vi "Test Elapsed Time.vi"() -> ()   [LabVIEW 2021, in "Interval Timer.lvlib"]
uses:
  Interval Timer.lvlib
panel:
  out "elapsed time (s)":dbl
  out "start time":timestamp
  out "current time":timestamp
  in  "wait (ms)":dbl=1000.0
  in  "reset?":bool
  in  "stop":bool
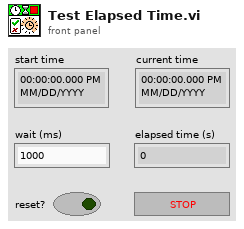
[diagram p1: front panel]
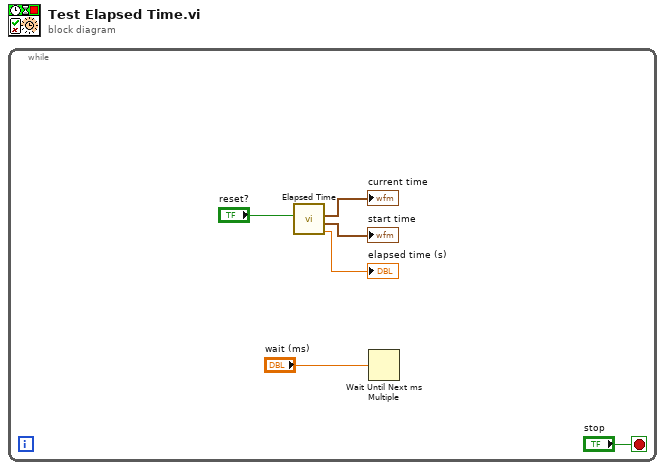
[diagram p0: block diagram]
diagram:
  n1 = while {
    stop <- "stop" stop-if-true
    n2 = call "Elapsed Time.vi"("reset timer"="reset?") -> ("elapsed time (s)"=→"elapsed time (s)":dbl, "start time"=→"start time":timestamp, "current time"=→"current time":timestamp)  [unwired: 8 in]
    n3 = Wait Until Next ms Multiple(millisecond multiple="wait (ms)") -> ()  [unwired: 1 out]
  }
